vi "Generate Square Wave.vi"(10 "Duty Cycle (%)":dbl, 11 "PWM Frequency":dbl) -> (3 "signal out":waveform(dbl))   [LabVIEW 2014]
uses:
  <vilib>/measure/NI_MABase.lvlib
panel:
  out "error out":errorcluster
  in  "error in (no error)":errorcluster
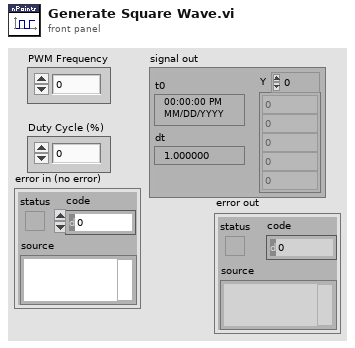
[diagram p1: front panel]
types:
  T1 = enum16{"Sine Wave", "Triangle Wave", "Square Wave", "Sawtooth Wave"}
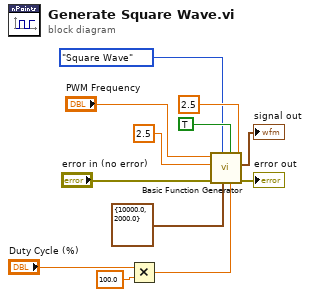
[diagram p0: block diagram]
diagram:
  n1 = Multiply(x="Duty Cycle (%)", y=100.0) -> (x*y=w1:dbl)
  n2 = call <vilib>:"Basic Function Generator.vi"("offset"=2.5, "square wave duty cycle (%)"=w1, "reset signal"=TRUE, "sampling info"=cluster{"Fs":dbl, "#s":dbl} {"Fs"=10000.0, "#s"=2000.0}, "signal type"=T1."Square Wave", "error in (no error)"="error in (no error)", "amplitude"=2.5, "frequency"="PWM Frequency") -> ("error out"=→"error out":errorcluster, "signal out"=→"signal out":waveform(dbl))  [unwired: 1 in, 1 out]
